vi "Cluster.vi"() -> ()   [LabVIEW 2018]
panel:
  out "결과":string
  out "출력 클러스터 2":cluster{"숫자":i32, "불리언":bool, "결과":string}
  out "출력 클러스터":cluster{i32, bool, string}
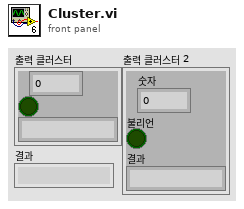
[diagram p1: front panel]
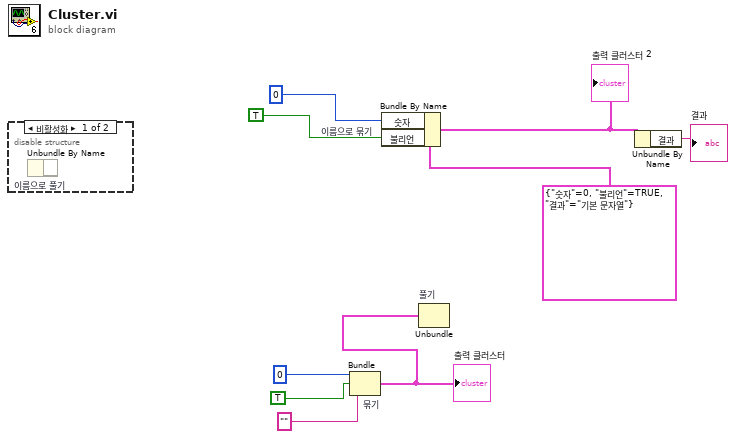
[diagram p0: block diagram]
diagram:
  n1 = disable-structure shown="비활성화" {
    frame Disabled {
      n2 = Unbundle By Name "이름으로 풀기"() -> ()  [unwired: 1 in, 1 out]
    }
    frame Enabled {
    }
  }
  n3 = Bundle "묶기"(0, TRUE, "") -> (w6:cluster{i32, bool, string})  [unwired: 1 in]
  "출력 클러스터" <- w6
  n4 = Bundle By Name "이름으로 묶기"(cluster=cluster{"숫자":i32, "불리언":bool, "결과":string} {"숫자"=0, "불리언"=TRUE, "결과"="기본 문자열"}, "숫자"=0, "불리언"=TRUE) -> (w2:cluster{"숫자":i32, "불리언":bool, "결과":string})
  "출력 클러스터 2" <- w2
  n5 = Unbundle "풀기"(w6) -> ()  [unwired: 3 out]
  n6 = Unbundle By Name(w2) -> ("결과"=→"결과":string)
